vi "OAT Torsional Vibration (Analog Tacho) (Even-Angle) (N Ch - N Settings).vi"(0 "analog tacho signals":waveform(dbl)[](array[waveform]), 1 "threshold (auto)":dbl[](array[numeric]), 2 "pulse/revolution (1)":i32[](array[numeric]) min=1, 3 "hysteresis (0)":dbl[](array[numeric]) format="%.2g", 4 "torsional vibration units":enum16{"RPM", "deg/s", "rad/s"}(ring), 5 "error in (no error)":errorcluster, 6 "missing pulses? (no:F)":bool[](array[boolean]), 7 "pulse width (2)":i32[](array[numeric]) min=0, 8 "reset? (F)":bool, 9 "slope (Rising)":u16[](array[ring]) items=["Rising", "Falling"]) -> (14 "even-angle torsional vibration signals":cluster{"r0":dbl, "dr":dbl, "Y":dbl[]}[](array[cluster]) {"r0" format="%.2p"; "dr" format="%.2p"; "Y" format="%.2f"}, 15 "even-angle channel info":T3[](array[typedef]) {"channel info"."pregain" format="%.2f"; "channel info"."weighting filter" items=["Linear", "A-weighting", "B-weighting", "C-weighting", "ITU-R 468-4", "Dolby", "CCITT", "C-message", "Wb", "Wc", "Wd", "We", "Wf", "Wh", "Wj", "Wk", "Wm", "AES17 20 kHz lowpass", "AES17 40 kHz lowpass", "AES17 20 kHz highpass", "AES17 40 kHz highpass"]; "channel info"."dB reference" format="%^.1e"; "channel info"."engineering units" items=["custom..."=0, "V"=1, "A"=21, "C"=30, "pC"=31, "s"=32, "-"=29, "Pa"=2, "N"=20, "g"=3, "m/s^2"=4, "m/s"=5, "m"=6, "mm/s"=12, "mm"=13, "micron/s"=14, "micron"=15, "in/s^2"=7, "in/s"=8, "in"=9, "mil/s"=10, "mil"=11, "rad/s^2"=16, "rad/s"=17, "rad"=18, "deg/s^2"=26, "deg/s"=27, "deg"=28, "RPM"=22, "cycle/s^2"=23, "Hz"=24, "cycle"=25, "strain"=19]; "channel info"."sensor sensitivity" format="%#_5f"}, 16 "speed profiles":T2[](array[typedef]) {"speed [RPM]" format="%.2f"; "time [s]" format="%.2f"}, 17 "position info":T1[](array[typedef]), 18 "unit labels":string[](array[string]), 19 "error out":errorcluster)   [LabVIEW 2017, in "SoundVib_Torsional.lvlib"]
doc: "Calculates torsional vibration signals from analog tachometer signals. This VI can return torsional vibration signals as either waveform signals or even-angle signals. Wire data to the <B>analog tacho signal</B> input to determine the polymorphic instance to use or manually select the instance."
uses:
  <vilib>/addons/Sound and Vibration/Order Analysis/Torsional Vibration/SoundVib_Torsional.lvlib
  <vilib>/addons/_NISVFA/_Shared subVIs/Controls/svc_Resampled Channel Info.ctl
  <vilib>/addons/_NISVFA/_Shared subVIs/Controls/svc_Channel Info.ctl
  <vilib>/addons/_NISVFA/_Shared subVIs/Controls/svc_Engineering Units Text Ring.ctl
  <vilib>/addons/_NISVFA/_Shared subVIs/Controls/svc_Weighting Filter Text Ring.ctl
  <vilib>/addons/Sound and Vibration/Order Analysis/Tach Process/SubVIs/speed profile.ctl
  <vilib>/addons/Sound and Vibration/Order Analysis/Misc/OAT Position Info.ctl
  <vilib>/addons/_NISVFA/_Shared subVIs/Common/svc_Check for Waveform Parameter Continuity (no state).vi
  <vilib>/addons/_NISVFA/_Shared subVIs/Common/svc_Get SV Channel Info.vi
  <vilib>/addons/_NISVFA/_Shared subVIs/Common/svc_Engineering Units to Unit Label.vi
  <vilib>/addons/_NISVFA/_Shared subVIs/Common/svc_Unit Label to Engineering Units.vi
  <vilib>/addons/Sound and Vibration/Order Analysis/Tach Process/SoundVib_TachProcess.lvlib
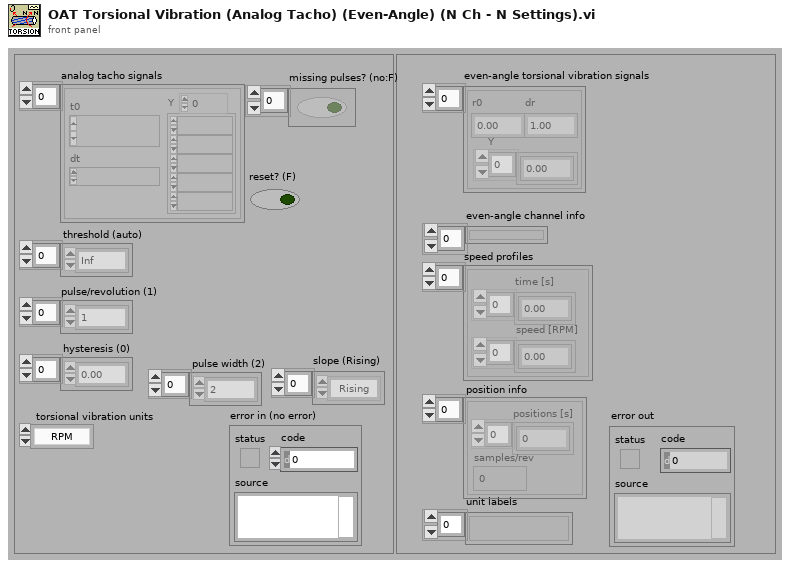
[diagram p1: front panel]
types:
  T1 = typedef "OAT Position Info.ctl" = cluster{"positions [s]":dbl[], "samples/rev":dbl}
  T2 = typedef "SoundVib_TachProcess.lvlib/speed profile.ctl" = cluster{"time [s]":dbl[], "speed [RPM]":dbl[]}
  T3 = typedef "svc_Resampled Channel Info.ctl" = cluster{"channel name":string, "description":string, " channel info":T4}
  T4 = typedef "svc_Channel Info.ctl" = cluster{"sensor sensitivity":dbl, "engineering units":T5, "dB reference":dbl, "custom label":string, "weighting filter":T6, "pregain":dbl}
  T5 = typedef "svc_Engineering Units Text Ring.ctl" = u16
  T6 = typedef "svc_Weighting Filter Text Ring.ctl" = u16
  T7 = cluster{"dt equal":bool, "array length equal":bool, "number channels change":bool}
  T8 = cluster{"dt":bool, "t0 continuity":bool, "array length":bool, "channel info":bool, "name":bool}
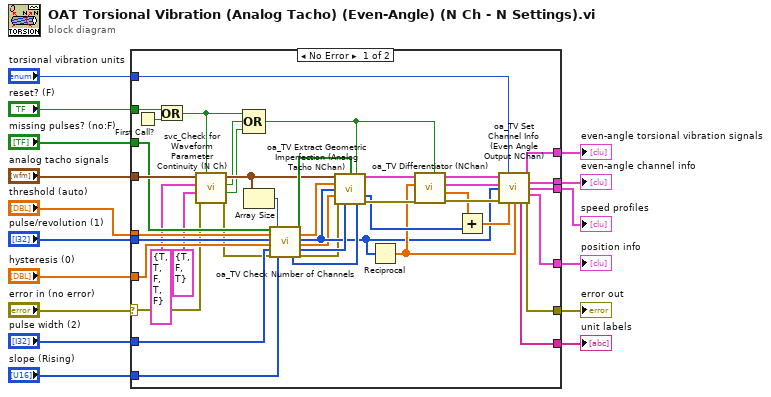
[diagram p0: block diagram]
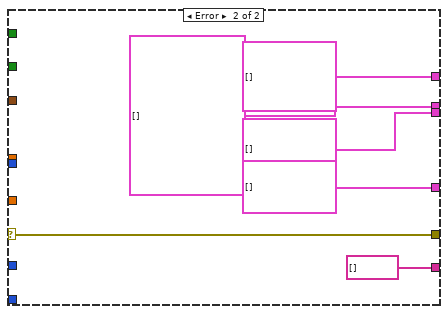
[diagram p2: hidden frame]
diagram:
  n1 = case shown="No Error" "error in (no error)" {
    selector: "error in (no error)" -> [w20 w64]
    tunnel: "threshold (auto)" -> [w51 _]
    tunnel: "pulse/revolution (1)" -> [w29 _]
    tunnel: "pulse width (2)" -> [w50 _]
    tunnel: "slope (Rising)" -> [w49 _]
    tunnel: "hysteresis (0)" -> [w28 _]
    tunnel: [w44 w64] -> w12
    tunnel: "reset? (F)" -> [w56 _]
    tunnel: "analog tacho signals" -> [w53 _]
    tunnel: [w40 cluster{"r0":dbl, "dr":dbl, "Y":dbl[]}[] []] -> w6
    tunnel: "torsional vibration units" -> [w38 _]
    tunnel: [w39 T3[] [] ("even-angle channel info")] -> w8
    tunnel: [w36 string[] [] ("unit labels")] -> w4
    tunnel: [w33 T2[] [] ("speed profiles")] -> w3
    tunnel: [w32 T1[] [] ("position info")] -> w2
    tunnel: "missing pulses? (no:F)" -> [w31 _]
    frame No Error {
      n2 = First Call?() -> (First Call?: T/F=w57:bool)
      n3 = Or(x=w56, y=w57) -> (x .or. y?=w24:bool)
      n4 = call <vilib>:"svc_Check for Waveform Parameter Continuity (N Ch).vi"("restart averaging (F)"=w24, "error in (no error)"=w20, "checks for multichannel parameters"=T7 {"dt equal"=TRUE, "array length equal"=FALSE, "number channels change"=TRUE}, "checks for channel parameter change"=T8 {"dt"=TRUE, "t0 continuity"=TRUE, "array length"=FALSE, "channel info"=TRUE, "name"=FALSE}, "scaled signal(s)"=w53) -> ("error out"=w19:errorcluster, "multichannel parameter changed"=w21:bool, "waveform parameter changed"=w22:bool, "dup scaled signal(s)"=w25:waveform(dbl)[])  [unwired: 3 out]
      n5 = Compound Arithmetic op=OR(w24, w22, w21) -> (w23:bool)
      n6 = Array Size(array=w25) -> (size(s)=w52:i32)
      n7 = call <vilib>:"oa_TV Check Number of Channels.vi"("missing pulses? (no:F)"=w31, "threshold (auto)"=w51, "pulse/revolution (1)"=w29, "hysteresis (0)"=w28, "pulse width (2)"=w50, "error in (no error)"=w19, "channel number"=w52, "slope (Rising)"=w49) -> ("slope out"=w46:u16[], "missing pulses? out"=w48:bool[], "threshold out"=w47:dbl[], "pulse/revolution out"=w34:i32[], "hysteresis out"=w27:dbl[], "pulse width out"=w37:i32[], "error out"=w30:errorcluster)  [unwired: 5 in]
      n8 = call <vilib>:"oa_TV Extract Geometric Imperfection (Analog Tacho NChan).vi"("analog tacho signal"=w25, "missing pulses? (no:F)"=w48, "reset? (F)"=w23, "threshold (auto)"=w47, "pulse/revolution"=w34, "hysteresis(0)"=w27, "error in (no error)"=w30, "pulse width (2)"=w37, "slope (Rising)"=w46) -> ("pulse positions"=w54:cluster{dbl[]}[], "revulotion index"=w55:i32[], "error out"=w58:errorcluster)  [unwired: 3 in, 1 out]
      n9 = Reciprocal(x=w34) -> (1/x=w43:dbl[])
      n10 = call <vilib>:"oa_TV Differentiator (NChan).vi"("reset? (False)"=w23, "error in (no error)"=w58, "delta X"=w43, "Y[n]"=w54) -> ("error out"=w45:errorcluster, "Delay"=w26:dbl[], "X[n]"=w35:cluster{dbl[]}[], "dY[n]/dX[n]"=w41:cluster{dbl[]}[])  [unwired: 4 in]
      n11 = Add(x=w26, y=w55) -> (x+y=w42:dbl[])
      n12 = call <vilib>:"oa_TV Set Channel Info (Even Angle Output NChan).vi"("seconds/revolution"=w41, "torisional vibration unit (RPM)"=w38, "pulse positions"=w35, "pulse/revolution (1)"=w34, "error in (no error)"=w45, "r0"=w42, "dr"=w43) -> ("even-angle torsional vibration"=w40:cluster{"r0":dbl, "dr":dbl, "Y":dbl[]}[], "even-angle channel info"=w39:T3[], "speed profiles"=w33:T2[], "position info"=w32:T1[], "unit labels"=w36:string[], "error out"=w44:errorcluster)  [unwired: 3 in]
    }
    frame Error {
    }
  }
  "error out" <- w12
  "even-angle channel info" <- w8
  "even-angle torsional vibration signals" <- w6
  "unit labels" <- w4
  "speed profiles" <- w3
  "position info" <- w2
